vi "TEST_SampleHanlder_move.vi"() -> ()   [LabVIEW 2017]
uses:
  <vilib>/Instr/_visa.llb/VISA Configure Serial Port (Instr).vi
panel:
  out "文字列":string
  in  "VISAリソース名":refnum<visa-resource-name>
  in  "停止":bool
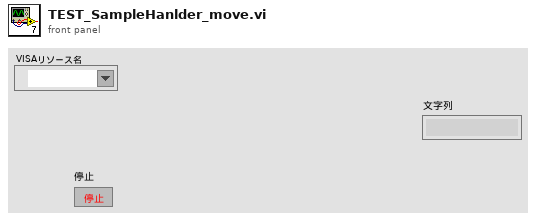
[diagram p1: front panel]
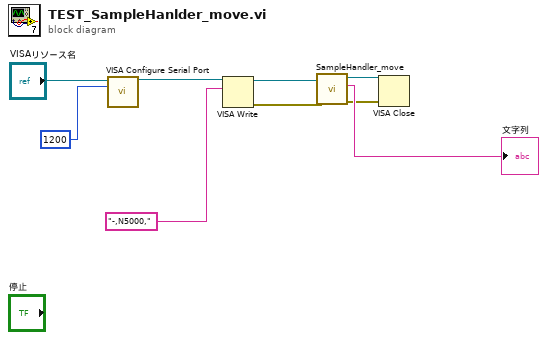
[diagram p0: block diagram]
diagram:
  n1 = call-poly "VISA Configure Serial Port"("VISA resource name"="VISAリソース名", "baud rate (9600)"=1200) -> ("VISA resource name out"=w8:refnum<visa-resource-name>)  [unwired: 12 in, 1 out]
  n2 = VISA Write(VISA resource name=w8, write buffer="-,N5000,") -> (VISA resource name out=w4:refnum<visa-resource-name>, error out=w5:errorcluster)  [unwired: 1 in, 1 out]
  n3 = call "SampleHandler_move.vi"("error in (no error)"=w5, "VISAリソース名"=w4) -> ("error out"=w1:errorcluster, "停止状態"=→"文字列":string, "VISAリソース名出力"=w2:refnum<visa-resource-name>)  [unwired: 7 in]
  n4 = VISA Close(VISA resource name=w2, error in (no error)=w1) -> ()  [unwired: 1 out]
